vi "HistogramAndFit.vi"(10 "Array":i32[](array[numeric])) -> (2 "Waveform Graph":dynamicdata(graph))   [LabVIEW 2014]
doc: "This program takes an array of data and creates a histogram. It also computes a best fit of the poisson distribution for the histogram\n\nBryan Ghahremani - SID: 1135515\nKenneth Heide - SID: 1269429"
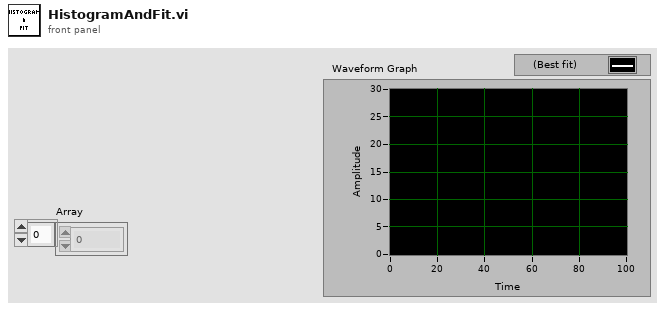
[diagram p1: front panel]
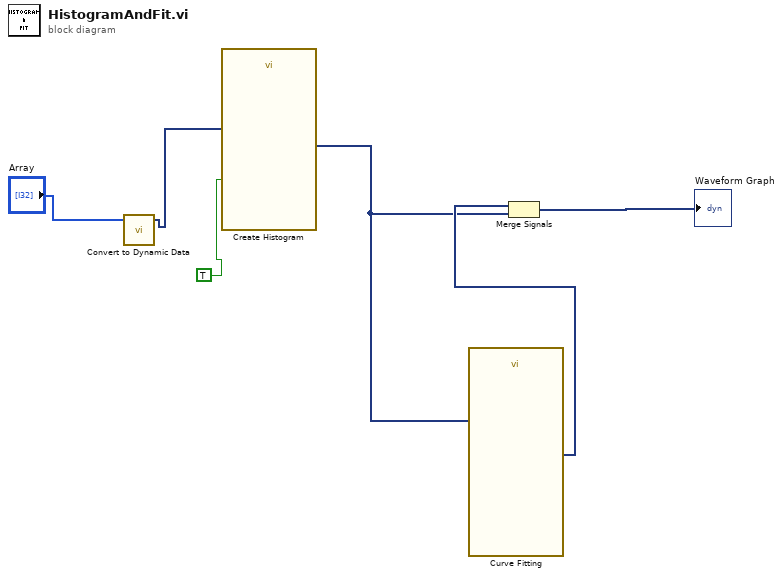
[diagram p0: block diagram]
diagram:
  n1 = call "Convert to Dynamic Data"("Array"="Array") -> ("Dynamic Data Type"=w3:dynamicdata)  [unwired: 3 in]
  n2 = call "Create Histogram"("Enable"=TRUE, "Signal"=w3) -> ("Histogram"=w5:dynamicdata)  [unwired: 8 in, 1 out]
  n3 = call "Curve Fitting"("Signals"=w5) -> ("best fit"=w6:dynamicdata)  [unwired: 6 in, 4 out]
  n4 = Merge Signals(w6, w5) -> (→"Waveform Graph":dynamicdata)
